vi "ClipModels.vi"(10 "Clip Plane State":enum16{"Inherit Value", "Off", "On"}(ring), 11 "Z":dbl) -> ()   [LabVIEW 2014]
uses:
  <vilib>/picture/3D Picture Control/Helpers/Set Clip Plane (no reference).vi
  <vilib>/picture/3D Picture Control/NI_3D Picture Control.lvlib
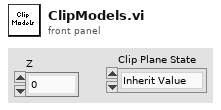
[diagram p1: front panel]
types:
  T1 = enum16{"New", "Find", "FindPattern", "GetTable", "Clear"}
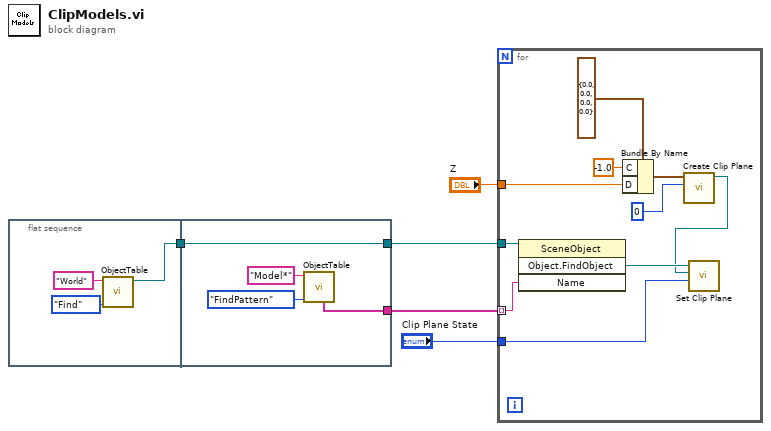
[diagram p0: block diagram]
diagram:
  n1 = flat-sequence {
    tunnel: [w6] -> w4
    tunnel: [w10] -> w5
    tunnel: w4 -> [w10]
    tunnel: [w9] -> w3
    frame #0 {
      n2 = call "ObjectTable.vi"("ObjectStoreSelector"=T1."Find", "Name"="World") -> ("ObjectRef"=w6:refnum<vi>)  [unwired: 5 in, 4 out]
    }
    frame #1 {
      n3 = call "ObjectTable.vi"("ObjectStoreSelector"=enum16{"New", "Find", "FindPattern", "GetTable"}."FindPattern", "Name"="Model*") -> ("Names"=w9:string[])  [unwired: 5 in, 4 out]
    }
  }
  n4 = for {
    tunnel: w5 -> [w22]
    tunnel: w3 -> [w21] mode=indexing
    tunnel: "Clip Plane State" -> [w19]
    tunnel: "Z" -> [w14]
    n5 = invoke class="SceneObject" method="Object.FindObject"(reference=w22, "Name"=w21) -> ("FindObject"=w20:refnum<vi>)  [unwired: 2 in, 3 out]
    n6 = Bundle By Name(cluster=cluster{"A":sgl, "B":sgl, "C":sgl, "D":sgl} {"A"=0.0, "B"=0.0, "C"=0.0, "D"=0.0} ("Plane"), "C"=sgl -1.0, "D"=w14) -> (w17:cluster{"A":sgl, "B":sgl, "C":sgl, "D":sgl})
    n7 = call <vilib>:"Create Clip Plane.vi"("Number"=0, "Plane"=w17) -> ("New Clip Plane Refnum"=w13:refnum<vi>)  [unwired: 8 in, 1 out]
    n8 = call-poly <vilib>:"Set Clip Plane.vi"("Clip Plane State"=w19, "Clip Plane Refnum In"=w13, "Scene Object In"=w20) -> ()  [unwired: 7 in, 2 out]
  }
